vi "FileIO-Jagged 2D Array to Spreadsheet String.vi"(0 "seqVals":dbl[](array[numeric]), 5 "spectra":cluster{"Freq":dbl[], "Mag":dbl[][]}[](array[cluster])) -> (4 "spreadsheet string":string)   [LabVIEW 2020]
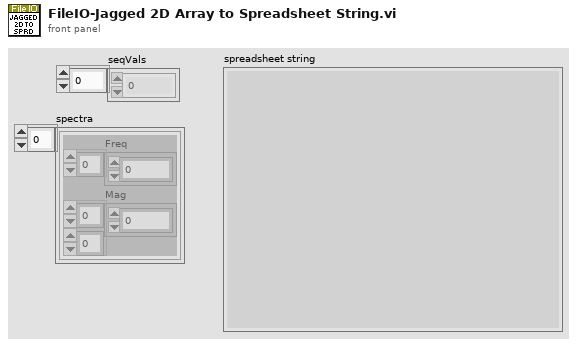
[diagram p1: front panel]
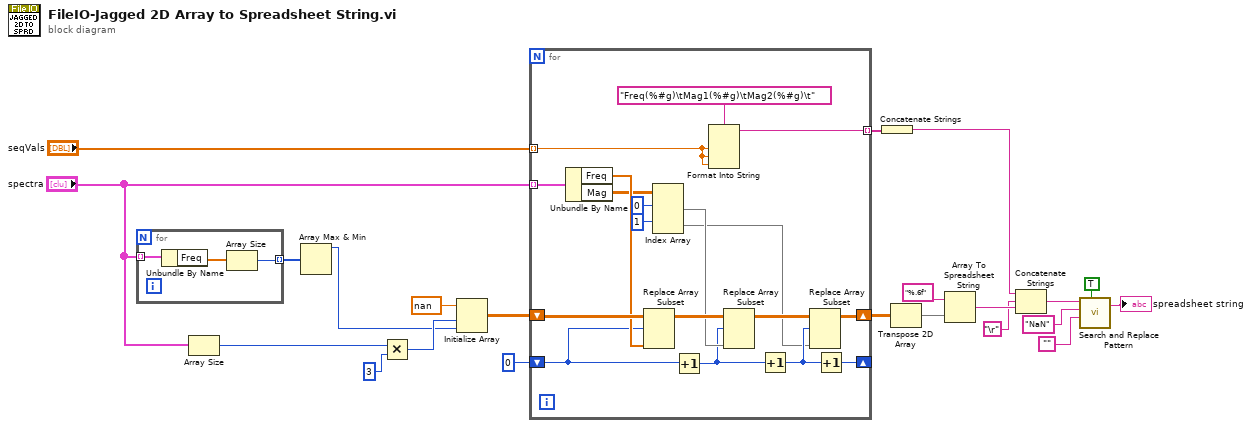
[diagram p0: block diagram]
diagram:
  n1 = for {
    tunnel: "spectra" -> [w25] mode=indexing
    tunnel: [w23] -> w22 mode=indexing
    n2 = Unbundle By Name(w25) -> ("Freq"=w24:dbl[])
    n3 = Array Size(array=w24) -> (size(s)=w23:i32)
  }
  n4 = Array Size(array="spectra") -> (size(s)=w21:i32)
  n5 = Array Max & Min(array=w22) -> (max value=w18:i32)  [unwired: 3 out]
  n6 = Multiply(x=w21, y=3) -> (x*y=w19:i32)
  n7 = Initialize Array(nan, w19, w18) -> (w15:dbl[][])
  n8 = for {
    tunnel: "spectra" -> [w43] mode=indexing
    shift-right: [w32] -> w13
    shift-left: w15 -> [w42]
    shift-right: [w26] -> _
    shift-left: 0 -> [w38]
    tunnel: "seqVals" -> [w30] mode=indexing
    tunnel: [w29] -> w9 mode=indexing
    n9 = Unbundle By Name(w43) -> ("Freq"=w41:dbl[], "Mag"=w40:dbl[][])
    n10 = Replace Array Subset(array=w42, new element=w41, index (row)=w38) -> (w39:dbl[][])  [unwired: 1 in]
    n11 = Index Array(array=w40, index (row) #1=0 ("index (row)"), index (row) #2=1 ("index (row)")) -> (element #1=w37:dbl[], element #2=w33:dbl[])  [unwired: 2 in]
    n12 = Increment(x=w38) -> (x+1=w36:i32)
    n13 = Format Into String(format string="Freq(%#g)\tMag1(%#g)\tMag2(%#g)\t", w30, w30, w30) -> (resulting string=w29:string)  [unwired: 2 in, 1 out]
    n14 = Replace Array Subset(array=w39, new element=w37, index (row)=w36) -> (w34:dbl[][])  [unwired: 1 in]
    n15 = Increment(x=w36) -> (x+1=w35:i32)
    n16 = Replace Array Subset(array=w34, new element=w33, index (row)=w35) -> (w32:dbl[][])  [unwired: 1 in]
    n17 = Increment(x=w35) -> (x+1=w26:i32)
  }
  n18 = Concatenate Strings(w9) -> (w7:string)
  n19 = Transpose 2D Array(2D array=w13) -> (transposed array=w12:dbl[][])
  n20 = Array To Spreadsheet String(array=w12, 3:"%.6f" ("format string")) -> (spreadsheet string=w8:string)  [unwired: 1 in]
  n21 = Concatenate Strings(w7, "\r", w8) -> (w5:string)
  n22 = call <vilib>:"Search and Replace Pattern.vi"("string"=w5, "regular expression (\"\")"="NaN" ("regular expression (\"\")"), "replace string (\"\")"="" ("replace string (\"\")"), "replace all? (F)"=TRUE) -> ("result string"=→"spreadsheet string":string)  [unwired: 1 in, 1 out]
